vi "Change_Graph_Scale_To_Log_vs_Log.vi"(8 "error in (no error)":errorcluster, 11 "Variant":variant) -> (0 "error out":errorcluster, 3 "data":variant)   [LabVIEW 2025]
uses:
  controls/Design_Results.ctl
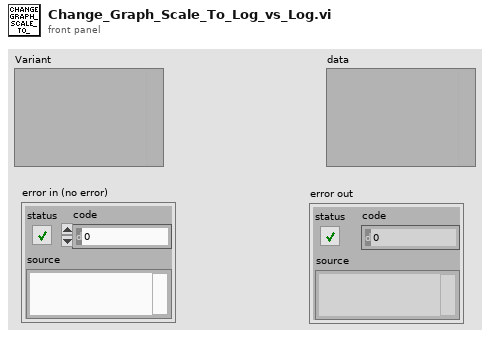
[diagram p1: front panel]
types:
  T1 = typedef "Design_Results.ctl" = cluster{"Design Results":cluster{"Model Validation: Simulated vs. Empirical Airflow Data":cluster{dbl[], dbl[]}[], "Amplitude - Empirical":string, "Power - Empirical":string, "Amplitude - Sim":string, "Power - Sim":string, "Flow Type":u32, "Optimized Inlet \nOrifice Diameter (in)":dbl, "Flow Type Name":string}}
  T2 = cluster{"sigma_delta_p_tap":dbl[], "m_dot":dbl[]}
  T3 = cluster{"sigma_delta_p_total":dbl[], "m_dot":dbl[]}
  T4 = cluster{"sigma_delta_p_empirical":dbl[], "m_dot":dbl[]}
  T5 = cluster{"sigma_delta_p_tap":dbl[], "m_dot":dbl[]}[]
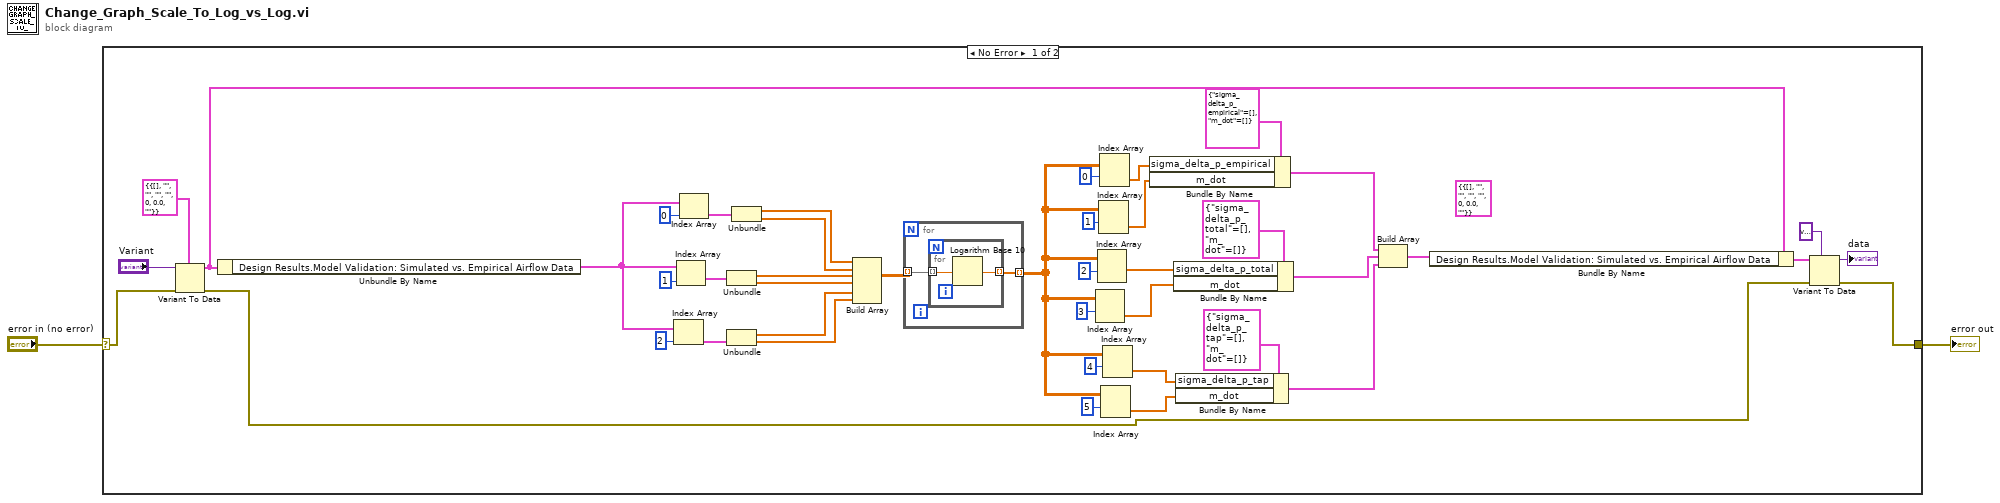
[diagram p0: block diagram]
diagram:
  n1 = case shown="No Error" "error in (no error)" {
    selector: "error in (no error)" -> [w6 w50]
    tunnel: [w4 w50] -> w1
    frame No Error {
      (unwired) T1 {"Design Results"={"Model Validation: Simulated vs. Empirical Airflow Data"=[], "Amplitude - Empirical"="", "Power - Empirical"="", "Amplitude - Sim"="", "Power - Sim"="", "Flow Type"=0, "Optimized Inlet \nOrifice Diameter (in)"=0.0, "Flow Type Name"=""}} ("data")
      n2 = Variant To Data(error in=w6, type=T1 {"Design Results"={"Model Validation: Simulated vs. Empirical Airflow Data"=[], "Amplitude - Empirical"="", "Power - Empirical"="", "Amplitude - Sim"="", "Power - Sim"="", "Flow Type"=0, "Optimized Inlet \nOrifice Diameter (in)"=0.0, "Flow Type Name"=""}} ("data"), Variant="Variant") -> (data=w3:T1, error out=w5:errorcluster)
      n3 = Unbundle By Name(w3) -> ("Design Results.Model Validation: Simulated vs. Empirical Airflow Data"=w20:cluster{dbl[], dbl[]}[])
      n4 = Index Array(array=w20, index=2 ("disabled index (col)")) -> (element=w24:cluster{dbl[], dbl[]})
      n5 = Index Array(array=w20, index=1 ("disabled index (col)")) -> (element=w22:cluster{dbl[], dbl[]})
      n6 = Index Array(array=w20, index=0 ("disabled index (col)")) -> (element=w21:cluster{dbl[], dbl[]})
      n7 = Unbundle(w22) -> (w31:dbl[], w32:dbl[])
      n8 = Unbundle(w24) -> (w33:dbl[], w34:dbl[])
      n9 = Unbundle(w21) -> (w23:dbl[], w30:dbl[])
      n10 = Build Array(w23, w30, w31, w32, w33, w34) -> (w25:dbl[][])
      n11 = for {
        tunnel: w25 -> [w47] mode=indexing
        tunnel: [w46] -> w43 mode=indexing
        n12 = for {
          tunnel: w47 -> [w48] mode=indexing
          tunnel: [w49] -> w46 mode=indexing
          n13 = Logarithm Base 10(1:w48) -> (0:w49:dbl)
        }
      }
      n14 = Index Array(array=w43, index (row)=3 ("disabled index (col)")) -> (element=w39:dbl[])  [unwired: 1 in]
      n15 = Index Array(array=w43, index (row)=2 ("disabled index (col)")) -> (element=w38:dbl[])  [unwired: 1 in]
      n16 = Index Array(array=w43, index (row)=1 ("disabled index (col)")) -> (element=w35:dbl[])  [unwired: 1 in]
      n17 = Index Array(array=w43, index (row)=0 ("disabled index (col)")) -> (element=w29:dbl[])  [unwired: 1 in]
      n18 = Index Array(array=w43, index (row)=5 ("disabled index (col)")) -> (element=w45:dbl[])  [unwired: 1 in]
      n19 = Index Array(array=w43, index (row)=4 ("disabled index (col)")) -> (element=w44:dbl[])  [unwired: 1 in]
      n20 = Bundle By Name(cluster=T4 {"sigma_delta_p_empirical"=[], "m_dot"=[]}, "sigma_delta_p_empirical"=w29, "m_dot"=w35) -> (w13:T4)
      n21 = Bundle By Name(cluster=T3 {"sigma_delta_p_total"=[], "m_dot"=[]}, "sigma_delta_p_total"=w38, "m_dot"=w39) -> (w12:T3)
      n22 = Bundle By Name(cluster=T2 {"sigma_delta_p_tap"=[], "m_dot"=[]}, "sigma_delta_p_tap"=w44, "m_dot"=w45) -> (w11:T2)
      n23 = Build Array(w13, w12, w11) -> (w10:T5)
      n24 = Bundle By Name(cluster=w3, "Design Results.Model Validation: Simulated vs. Empirical Airflow Data"=w10) -> (w8:T1)
      n25 = Variant To Data(error in=w5, type=variant ("Variant"), Variant=w8) -> (data=→"data":variant, error out=w4:errorcluster)
    }
    frame Error {
    }
  }
  "error out" <- w1
